vi "LoadConfigurationFromSetupMemory.vi"(2 "error in (no error)":errorcluster, 3 "Configuration Name":string, 4 "Load Configuration from Setup Memory":u16(ring) items=["Memory 0", "Memory 1", "Memory 2", "Memory 3", "Memory 4", "Configuration"], 5 "VISA resource name":refnum<visa-resource-name>) -> (0 "error out":errorcluster, 1 "VISA resource name out":refnum<visa-resource-name>)   [LabVIEW 2020, in "Active Technologies AWG3000.lvlib"]
uses:
  Active Technologies AWG3000.lvlib
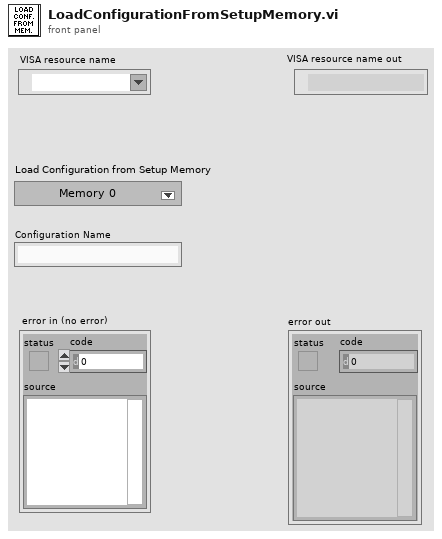
[diagram p1: front panel]
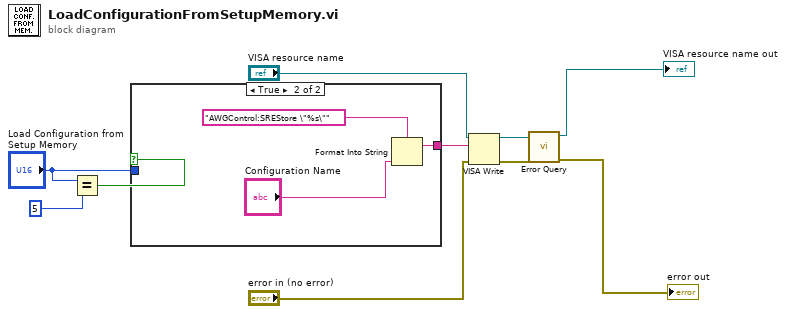
[diagram p0: block diagram]
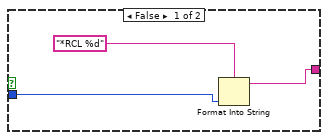
[diagram p2: hidden frame]
diagram:
  n1 = Equal?(x="Load Configuration from Setup Memory", y=u16 5) -> (x = y?=w2:bool)
  n2 = case shown="True" w2 {
    tunnel: [w11 w16] -> w8
    tunnel: "Load Configuration from Setup Memory" -> [w12 _]
    frame False {
      n3 = Format Into String(format string="*RCL %d" ("write buffer"), w12) -> (resulting string=w11:string)  [unwired: 2 in, 1 out]
    }
    frame True {
      n4 = Format Into String(format string="AWGControl:SREStore \"%s\"" ("write buffer"), "Configuration Name") -> (resulting string=w16:string)  [unwired: 2 in, 1 out]
    }
  }
  n5 = VISA Write(VISA resource name="VISA resource name", write buffer=w8, error in (no error)="error in (no error)") -> (VISA resource name out=w7:refnum<visa-resource-name>, error out=w6:errorcluster)  [unwired: 1 out]
  n6 = call "Error Query.vi"("error in (no error)"=w6, "VISA resource name"=w7) -> ("error out"=→"error out":errorcluster, "VISA resource name out"=→"VISA resource name out":refnum<visa-resource-name>)  [unwired: 6 in, 2 out]
